vi "Get Attributes Name.vi"(8 "error in (no error)":errorcluster, 11 "YAML Parser in":refnum<class "YAML Parser.lvclass">) -> (0 "error out":errorcluster, 1 "Count":i32, 2 "Attributes":string[](array[string]), 3 "YAML Parser out":refnum<class "YAML Parser.lvclass">)   [LabVIEW 2015, in "YAML Parser.lvclass"]
uses:
  YAML Parser.lvclass
  YAML Parser.lvclass/YAML Parser.ctl
  <vilib>/Utility/error.llb/Error Cluster From Error Code.vi
  <vilib>/ErrorRing/Error Ring.xnode
  <vilib>/Utility/Data Type/NI_Data Type.lvlib
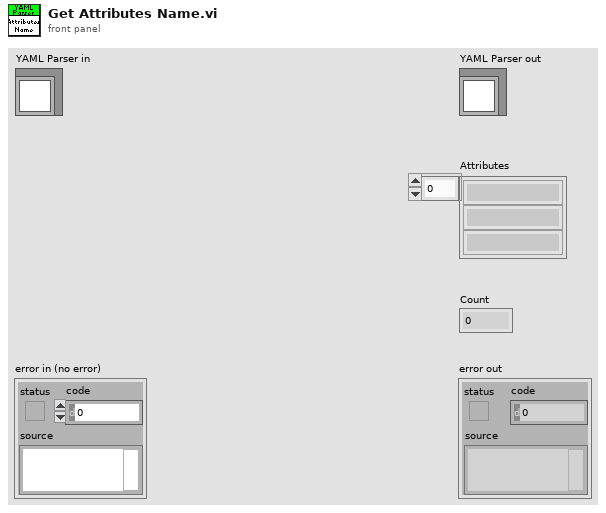
[diagram p1: front panel]
types:
  T1 = typedef "NI_Data Type.lvlib/Data Type.ctl" = enum8{"Invalid Type", "Void", "I8", "I16", "I32", "I64", "U8", "U16", "U32", "U64", "Single Float", "Double Float", "Extended Float", "Single Complex", "Double Complex", "Extended Complex", "Enum U8", "Enum U16", "Enum U32", "Enum U64", "Single Float With Unit", "Double Float With Unit", "Extended Float With Unit", "Single Complex with Unit", "Double Complex with Unit", "Extended Complex with Unit", "Boolean", "String", "Path", "Picture", "Tag", "Array", "Cluster", "Variant", "LV Variant", "Waveform", "Timestamp", "Digital Waveform", "Digital Data", "ExpressData", "Refnum", "External Data", "VI", "Poly VI", "LabVIEW Class Instance", "Fixed Point"}
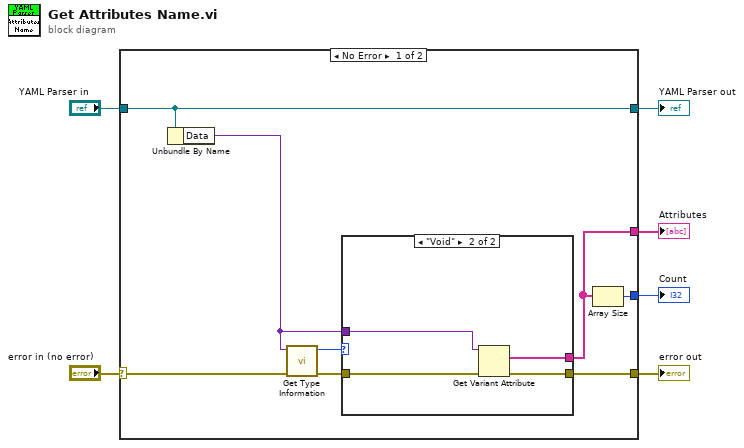
[diagram p0: block diagram]
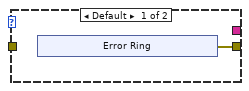
[diagram p2: hidden frame]
diagram:
  n1 = case shown="No Error" "error in (no error)" {
    selector: "error in (no error)" -> [w13 w26]
    tunnel: [w10 w26] -> w5
    tunnel: [w14 w25] -> w3
    tunnel: "YAML Parser in" -> [w14 w25]
    tunnel: [w8 _] -> w2
    tunnel: [w7 _] -> w1
    frame No Error {
      n2 = Unbundle By Name(w14) -> ("Data"=w9:variant)
      n3 = call <vilib>:"Get Type Information.vi"("error in (no error)"=w13, "Variant"=w9) -> ("error out"=w12:errorcluster, "Type"=w11:T1)  [unwired: 5 in, 3 out]
      n4 = case shown="\"Void\"" w11 {
        tunnel: w12 -> [_ w24]
        tunnel: [w15 w22] -> w10
        tunnel: w9 -> [_ w23]
        tunnel: [_ w21] -> w8
        frame Default {
          n5 = xnode "Error Ring"() -> ("error out"=w15:errorcluster)
        }
        frame "Void" {
          n6 = Get Variant Attribute(Variant=w23, error in=w24) -> (names=w21:string[], error out=w22:errorcluster)  [unwired: 2 in, 2 out]
        }
      }
      n7 = Array Size(array=w8) -> (size(s)=w7:i32)
    }
    frame Error {
    }
  }
  "error out" <- w5
  "YAML Parser out" <- w3
  "Count" <- w1
  "Attributes" <- w2
